vi "CleanUp.vi"(0 "object in":refnum<class "Stack.lvclass">, 11 "Error In":errorcluster) -> (4 "object out":refnum<class "Stack.lvclass">, 15 "Error Out":errorcluster)   [LabVIEW 2024, in "Stack.lvclass"]
uses:
  Stack.lvclass
  Stack.lvclass/Stack.ctl
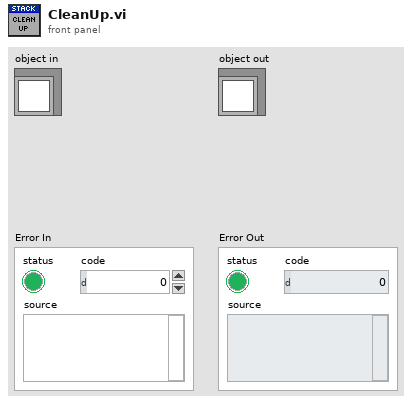
[diagram p1: front panel]
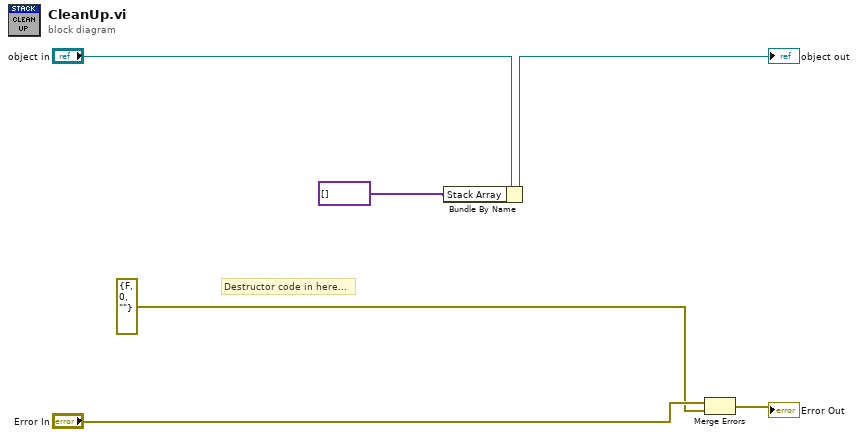
[diagram p0: block diagram]
diagram:
  # "Destructor code in here..."
  n1 = Bundle By Name(cluster="object in", "Stack Array"=variant[] []) -> (→"object out":refnum<class "Stack.lvclass">)
  n2 = Merge Errors("Error In", errorcluster {"status"=FALSE, "code"=0, "source"=""} ("error in (no error)")) -> (→"Error Out":errorcluster)
